vi "VI-Rename Project Items.vi"() -> (15 "error out":errorcluster)   [LabVIEW 2020]
panel:
  in  "Old prefix":string="EPT"
  in  "Prefix":string
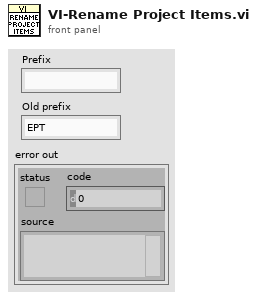
[diagram p1: front panel]
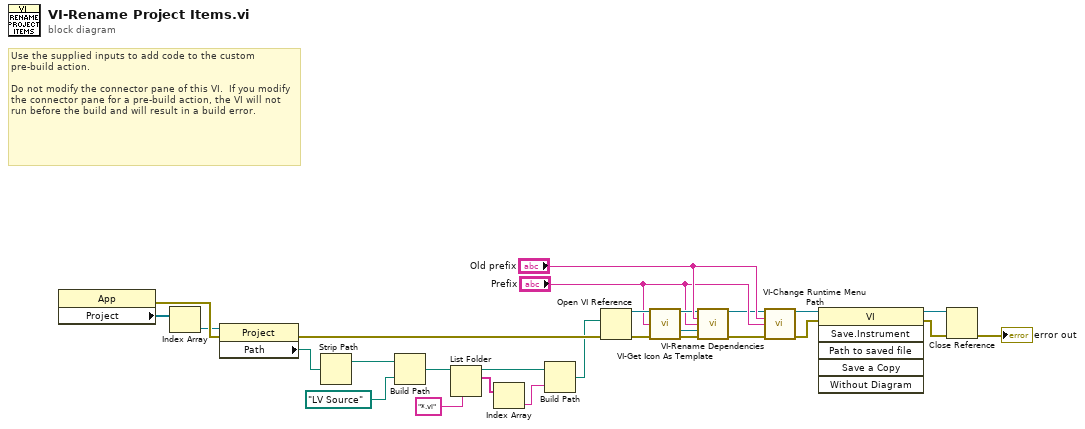
[diagram p0: block diagram]
diagram:
  # "Use the supplied inputs to add code to the custom pre-build action.\n\nDo not modify the connector pane of this VI.  If you modify the connector pane for a pre-build action, the VI will not run before the build and will result in a build error."
  n1 = property class="App"() -> (error out=w27:errorcluster, "Project"=w26:refnum<vi>[])  [unwired: 2 in, 1 out]
  n2 = Index Array(array=w26) -> (element=w25:refnum<vi>)  [unwired: 1 in]
  n3 = property class="Project"(reference=w25, error in=w27) -> (error out=w14:errorcluster, "Path"=w24:path)  [unwired: 1 out]
  n4 = Strip Path(path=w24) -> (stripped path=w23:path)  [unwired: 1 out]
  n5 = Build Path(base path=w23, name or relative path=path "LV Source") -> (appended path=w21:path)
  n6 = List Folder(path=w21, pattern="*.vi") -> (path out=w19:path, filenames=w18:string[])  [unwired: 2 in, 2 out]
  n7 = Index Array(array=w18) -> (element=w17:string)  [unwired: 1 in]
  n8 = Build Path(base path=w19, name or relative path=w17) -> (appended path=w13:path)
  n9 = Open VI Reference(vi path=w13, error in (no error)=w14) -> (vi reference=w10:refnum<vi>, error out=w7:errorcluster)  [unwired: 4 in]
  n10 = call "VI-Get Icon As Template.vi"("VIref in"=w10, "Prefix"="Prefix", "error in (no error)"=w7) -> ("VIref out"=w9:refnum<vi>, "Icon Framework.lvclass out"=w1:refnum<class "Icon Framework.lvclass">, "error out"=w8:errorcluster)  [unwired: 10 in]
  n11 = call "VI-Rename Dependencies.vi"("VIref in"=w9, "Old prefix"="Old prefix", "New prefix"="Prefix", "Icon Template"=w1, "error in (no error)"=w8) -> ("VIref out"=w4:refnum<vi>, "error out"=w5:errorcluster)  [unwired: 9 in]
  n12 = call "VI-Change Runtime Menu Path.vi"("VIref in"=w4, "Old prefix"="Old prefix", "New prefix"="Prefix", "error in (no error)"=w5) -> ("VIref out"=w3:refnum<vi>, "error out"=w2:errorcluster)  [unwired: 10 in]
  n13 = invoke class="VI" method="Save.Instrument"(reference=w3, error in=w2) -> (reference out=w16:refnum<vi>, error out=w15:errorcluster)  [unwired: 4 in, 4 out]
  n14 = Close Reference(reference=w16, error in (no error)=w15) -> (error out=→"error out":errorcluster)
